vi "Script Message Enqueuers Reference Components.vi"(8 "error in (no error)":errorcluster, 10 "Message Enqueuers to Add":T2[](array[typedef]), 11 "Message Enqueuer Component Paths":T1) -> (0 "error out":errorcluster)   [LabVIEW 2018, in "Scripting.lvlib"]
uses:
  Scripting.lvlib
  Error-Codes.ctl
  <vilib>/Utility/miscctls.llb/LVPositionTypeDef.ctl
  <vilib>/Utility/traverseref.llb/VI Scripting - Traverse.lvlib
  <vilib>/Utility/traverseref.llb/TRef TravTarget.ctl
  Event-Type-Information.ctl
  Message-Enqueuer Component Paths.ctl
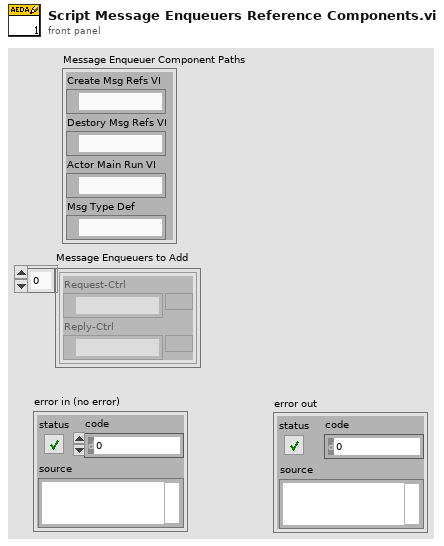
[diagram p1: front panel]
types:
  T1 = typedef "Scripting.lvlib/Message-Enqueuer Component Paths.ctl" = cluster{"Create Msg Refs VI":path, "Destory Msg Refs VI":path, "Actor Main Run VI":path, "Msg Type Def":path}
  T2 = typedef "Scripting.lvlib/Event-Type-Information.ctl" = cluster{"Request-Ctrl":path, "Reply-Ctrl":path}
  T3 = typedef "Scripting.lvlib/Error-Codes.ctl" = enum16{"EVENT_REF_TYPE_DEF_IS_NESTED", "EVENT_REF_TYPE_DEF_IS_EMPTY", "EVENT_REF_TYPE_DEF_INCLUDES_NON_REFS", "EVENT_REF_TYPE_INVALID_REPLY_REF", "EVENT_REF_TYPE_REPLY_IS_NOT_TYPE_DEF", "EVENT_REF_TYPE_DEF_IS_NOT_CLUSTER", "EVENT_REF_TYPE_DEF_INVALID_REQ_REPLY_TYPE", "ACTOR_CLASS_PATH_IS_INVALID", "ACTOR_CLASS_LIBRARY_IS_NOT_EDITABLE", "ACTOR_CLASS_CREATE_ENQUEUER_REFS_VI_NOT_FOUND", "MSG_ENQUEUER_REFS_CTL_NOT_FOUND", "ACTOR_CLASS_MAIN_RUN_VI_NOT_FOUND", "ACTOR_CLASS_DESTROY_ENQUEUER_REFS_VI_NOT_FOUND", "CREATE_ENQUEUER_REFS_ERROR_TERMINAL_NOT_FOUND", "CREATE_ENQUEUER_REFS_INVALID_TYPE_DEF", "CREATE_ENQUEUER_REF_NAMEBUNDLER_NOT_FOUND", "CREATE_ENQUEUER_REF_MULTIPLE_NAMEBUNDLERS"}
  T4 = typedef "TRef TravTarget.ctl" = enum16{"FP", "BD", "Other"}
  T5 = typedef "LVPositionTypeDef.ctl" = cluster{"Left":i32, "Top":i32}
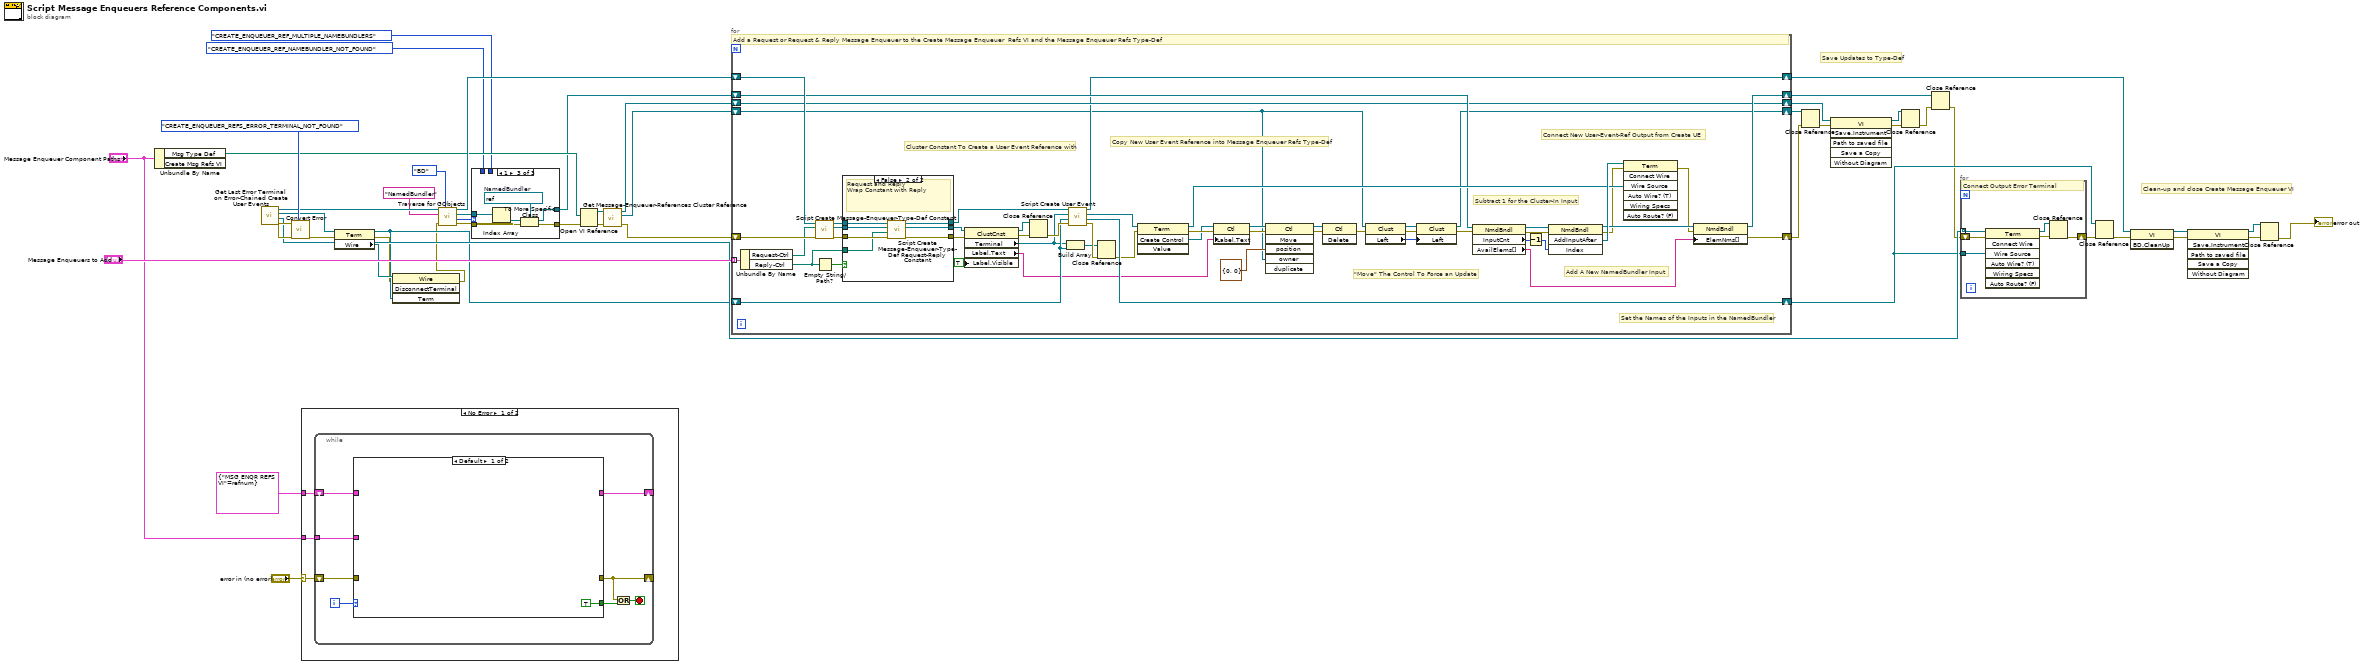
[diagram p0: block diagram]
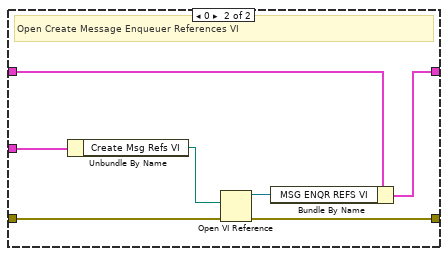
[diagram p2: hidden frame]
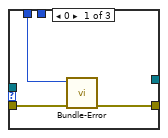
[diagram p4: hidden frame]
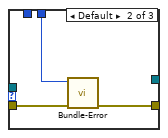
[diagram p5: hidden frame]
diagram:
  # "Clean-up and close Create Message Enqueuer VI"
  # "Save Updates to Type-Def"
  n1 = Unbundle By Name("Message Enqueuer Component Paths") -> ("Msg Type Def"=w40:path, "Create Msg Refs VI"=w48:path)
  n2 = call "Get Last Error Terminal on Error-Chained Create User Events.vi"() -> ("error out"=w46:errorcluster, "Connected Sink Terminals"=w29:refnum<vi>[], "Last Error Source Terminal"=w8:refnum<vi>, "VI out"=w44:refnum<vi>, "error in (no error)"=w45:errorcluster)  [unwired: 7 in]
  n3 = call "Convert Error.vi"("Convert to Error Code"=Error-Codes."CREATE_ENQUEUER_REFS_ERROR_TERMINAL_NOT_FOUND", "error in (no error)"=w45, "Error Input"=w46) -> ("error out"=w7:errorcluster)  [unwired: 8 in]
  n4 = case shown="No Error" "error in (no error)" {
    selector: "error in (no error)" -> [w52 _]
    tunnel: "Message Enqueuer Component Paths" -> [w53 _]
    tunnel: cluster{"MSG ENQR REFS VI":refnum<vi>} {"MSG ENQR REFS VI"=refnum} -> [w51 _]
    frame No Error {
      n5 = while {
        tunnel: w53 -> [w58]
        shift-right: [w54] -> _
        shift-left: w52 -> [w57]
        shift-right: [w55] -> _
        shift-left: w51 -> [w56]
        i -> [w61]
        stop <- w59 stop-if-true
        n6 = case shown="Default" w61 {
          tunnel: [TRUE _] -> w60
          tunnel: w58 -> [_ w69]
          tunnel: w57 -> [_ w68]
          tunnel: w56 -> [_ w66]
          tunnel: [_ w64] -> w55
          tunnel: [_ w63] -> w54
          frame Default {
          }
          frame 0 {
            # "Open Create Message Enqueuer References VI"
            n7 = Unbundle By Name(w69) -> ("Create Msg Refs VI"=w67:path)
            n8 = Open VI Reference(vi path=w67, error in (no error)=w68) -> (vi reference=w65:refnum<vi>, error out=w63:errorcluster)  [unwired: 4 in]
            n9 = Bundle By Name(cluster=w66, "MSG ENQR REFS VI"=w65) -> (w64:cluster{"MSG ENQR REFS VI":refnum<vi>})
          }
        }
        n10 = Or(x=w54, y=w60) -> (x .or. y?=w59:bool)
      }
    }
    frame Error {
    }
  }
  n11 = property class="Term"(reference=w8, error in=w7) -> (reference out=w6:refnum<vi>, error out=w5:errorcluster, "Wire"=w9:refnum<vi>)
  n12 = invoke class="Wire" method="DisconnectTerminal"(reference=w9, error in=w5, "Term"=w6) -> (error out=w4:errorcluster)  [unwired: 1 in, 3 out]
  n13 = call <vilib>:"Traverse for GObjects.vi"("Traverse Target"=TRef_TravTarget."BD", "error in (no error)"=w4, "Class Name"="NamedBundler", "VI Refnum"=w44) -> ("error out"=w30:errorcluster, "# of Refs"=w31:i32, "References"=w32:refnum<vi>[], "dup VI Refnum"=w42:refnum<vi>)  [unwired: 4 in]
  n14 = case shown="1" w31 {
    tunnel: w32 -> [_ _ w81]
    tunnel: w30 -> [w72 w75 w78]
    tunnel: [w71 w74 w77] -> w35
    tunnel: [_ _ w76] -> w36
    tunnel: Error-Codes."CREATE_ENQUEUER_REF_NAMEBUNDLER_NOT_FOUND" ("Errors") -> [w70 _ _]
    tunnel: Error-Codes."CREATE_ENQUEUER_REF_MULTIPLE_NAMEBUNDLERS" ("Errors") -> [_ w73 _]
    frame 0 {
      n15 = call "Bundle-Error.vi"("error in (no error)"=w72, "Errors"=w70) -> ("error out"=w71:errorcluster)  [unwired: 9 in]
    }
    frame Default {
      n16 = call "Bundle-Error.vi"("error in (no error)"=w75, "Errors"=w73) -> ("error out"=w74:errorcluster)  [unwired: 9 in]
    }
    frame 1 {
      w79 = refnum<vi> refnum  # NamedBundler
      n17 = Index Array(array=w81) -> (element=w80:refnum<vi>)  [unwired: 1 in]
      n18 = To More Specific Class(target class=w79, reference=w80, error in=w78) -> (specific class reference=w76:refnum<vi>, error out=w77:errorcluster)
    }
  }
  n19 = Open VI Reference(vi path=w40, error in (no error)=w35) -> (vi reference=w39:refnum<vi>, error out=w41:errorcluster)  [unwired: 4 in]
  n20 = call "Get Message-Enqueuer-References Cluster Reference.vi"("error in (no error)"=w41, "VI Refnum in"=w39) -> ("error out"=w43:errorcluster, "Cluster"=w38:refnum<vi>, "VI Refnum out"=w37:refnum<vi>)  [unwired: 7 in]
  n21 = for {
    shift-right: [w125] -> w27
    shift-left: w6 -> [w126]
    tunnel: "Message Enqueuers to Add" -> [w134] mode=indexing
    shift-right: [w102] -> w25
    shift-left: w43 -> [w100]
    shift-right: [w87] -> w26
    shift-left: w38 -> [w83]
    shift-right: [w86] -> w24
    shift-left: w37 -> [w86]
    shift-right: [w88] -> w19
    shift-left: w36 -> [w90]
    shift-right: [w85] -> w17
    shift-left: w42 -> [w97]
    # "Set the Names of the Inputs in the NamedBundler"
    # "Connect New User-Event-Ref Output from Create UE"
    # "Add A New NamedBundler Input"
    # "Subtract 1 for the Cluster-In Input"
    # "Copy New User Event Reference into Message Enqueuer Refs Type-Def"
    # "Cluster Constant To Create a User Event Reference with"
    # "\"Move\" The Control To Force an Update"
    # "Add a Request or Request & Reply Message Enqueuer to the Create Message Enqueuer  Refs VI and the Message Enqueuer Refs Type-Def"
    n22 = Unbundle By Name(w134) -> ("Request-Ctrl"=w96:path, "Reply-Ctrl"=w95:path)
    n23 = call "Script Create Message-Enqueuer-Type-Def Constant.vi"("error in (no error)"=w100, "Type-Def Path"=w96, "VI in"=w97) -> ("error out"=w99:errorcluster, "ClusterConstant"=w94:refnum<vi>, "VI out"=w98:refnum<vi>)  [unwired: 6 in]
    n24 = Empty String/Path?(string/path=w95) -> (empty?=w133:bool)
    n25 = case shown="False" w133 {
      tunnel: w98 -> [w135 w144]
      tunnel: w99 -> [w137 w143]
      tunnel: [w137 w138] -> w132
      tunnel: w95 -> [_ w142]
      tunnel: w94 -> [w136 w141]
      tunnel: [w136 w139] -> w93
      tunnel: [w135 w140] -> w92
      frame True {
        # "Request Only"
      }
      frame False {
        # "Request and Reply\nWrap Constant with Reply"
        n26 = call "Script Create Message-Enqueuer-Type-Def Request-Reply Constant.vi"("error in (no error)"=w143, "Reply-Ctrl"=w142, "Request Cluster Constant"=w141, "VI in"=w144) -> ("error out"=w138:errorcluster, "Request-Reply Cluster Constant"=w139:refnum<vi>, "VI out"=w140:refnum<vi>)  [unwired: 5 in]
      }
    }
    n27 = property class="ClustCnst"(reference=w93, error in=w132, "Label.Visible"=TRUE) -> (reference out=w130:refnum<vi>, error out=w131:errorcluster, "Terminal"=w91:refnum<vi>, "Label.Text"=w89:string)
    n28 = Close Reference(reference=w130, error in (no error)=w131) -> (error out=w129:errorcluster)
    n29 = Build Array(w91, w126) -> (w127:refnum<vi>[])
    n30 = call "Script Create User Event.vi"("error in (no error)"=w129, "Error In Sink Terminal"=w126, "User Event Data Constant Terminal"=w91, "VI in"=w92) -> ("error out"=w128:errorcluster, "Error Out Source Terminal"=w125:refnum<vi>, "User Event Reference Out Terminal"=w119:refnum<vi>, "VI out"=w85:refnum<vi>)  [unwired: 4 in]
    n31 = Close Reference(reference=w127, error in (no error)=w128) -> (error out=w118:errorcluster)
    n32 = invoke class="Term" method="Create Control"(reference=w119, error in=w118) -> (reference out=w111:refnum<vi>, error out=w117:errorcluster, "Create Control"=w116:refnum<vi>)  [unwired: 2 in, 1 out]
    n33 = property class="Ctl"(reference=w116, error in=w117, "Label.Text"=w89) -> (reference out=w124:refnum<vi>, error out=w123:errorcluster)
    n34 = invoke class="Ctl" method="Move"(reference=w124, error in=w123, "position"=T5 {"Left"=0, "Top"=0}, "owner"=w83) -> (reference out=w121:refnum<vi>, error out=w120:errorcluster)  [unwired: 2 in, 4 out]
    n35 = invoke class="Ctl" method="Delete"(reference=w121, error in=w120) -> (error out=w103:errorcluster)  [unwired: 1 in, 2 out]
    n36 = property class="Clust"(reference=w83, error in=w103) -> (reference out=w106:refnum<vi>, error out=w105:errorcluster, "Left"=w104:i32)
    n37 = property class="Clust"(reference=w106, error in=w105, "Left"=w104) -> (reference out=w87:refnum<vi>, error out=w101:errorcluster)
    n38 = property class="NmdBndl"(reference=w90, error in=w101) -> (reference out=w115:refnum<vi>, error out=w113:errorcluster, "InputCnt"=w114:i32, "AvailElems[]"=w84:string[])
    n39 = Decrement(x=w114) -> (x-1=w107:i32)
    n40 = invoke class="NmdBndl" method="AddInputAfter"(reference=w115, error in=w113, "Index"=w107) -> (reference out=w110:refnum<vi>, error out=w108:errorcluster, "AddInputAfter"=w112:refnum<vi>)  [unwired: 1 in, 1 out]
    n41 = invoke class="Term" method="Connect Wire"(reference=w112, error in=w108, "Wire Source"=w111) -> (error out=w109:errorcluster)  [unwired: 4 in, 6 out]
    n42 = property class="NmdBndl"(reference=w110, error in=w109, "ElemNms[]"=w84) -> (reference out=w88:refnum<vi>, error out=w102:errorcluster)
  }
  n43 = Close Reference(reference=w26, error in (no error)=w25) -> (error out=w23:errorcluster)
  n44 = invoke class="VI" method="Save.Instrument"(reference=w24, error in=w23) -> (reference out=w21:refnum<vi>, error out=w22:errorcluster)  [unwired: 4 in, 4 out]
  n45 = Close Reference(reference=w21, error in (no error)=w22) -> (error out=w20:errorcluster)
  n46 = Close Reference(reference=w19, error in (no error)=w20) -> (error out=w18:errorcluster)
  n47 = for {
    tunnel: w29 -> [w150] mode=indexing
    shift-right: [w146] -> w28
    shift-left: w18 -> [w149]
    tunnel: w27 -> [w145]
    # "Connect Output Error Terminal"
    n48 = invoke class="Term" method="Connect Wire"(reference=w150, error in=w149, "Wire Source"=w145) -> (reference out=w147:refnum<vi>, error out=w148:errorcluster)  [unwired: 4 in, 5 out]
    n49 = Close Reference(reference=w147, error in (no error)=w148) -> (error out=w146:errorcluster)
  }
  n50 = Close Reference(reference=w27, error in (no error)=w28) -> (error out=w13:errorcluster)
  n51 = invoke class="VI" method="BD.CleanUp"(reference=w17, error in=w13) -> (reference out=w14:refnum<vi>, error out=w12:errorcluster)  [unwired: 1 in, 1 out]
  n52 = invoke class="VI" method="Save.Instrument"(reference=w14, error in=w12) -> (reference out=w15:refnum<vi>, error out=w16:errorcluster)  [unwired: 4 in, 4 out]
  n53 = Close Reference(reference=w15, error in (no error)=w16) -> (error out=→"error out":errorcluster)
